vi "2. MotorTest.vi"(1 "Stop Button":bool, 8 "error in (no error)":errorcluster, 10 "Speed (PWM)":dbl(slide) scale=-100.0..100.0) -> (0 "error out":errorcluster, 2 "MotorEncoder (deg)":dbl)   [LabVIEW 2019, in "SJCube_KNRm.lvlib"]
uses:
  SJCube_KNRm.lvlib
panel:
  in  "Reset Counter":bool
  out "gearedMotorEncoder (deg)":dbl
  # "ATTENTION:\n\nDO THIS EXP. ONLY WHEN THE PENDULUM \nIS \"NOT\" INSTALLED"
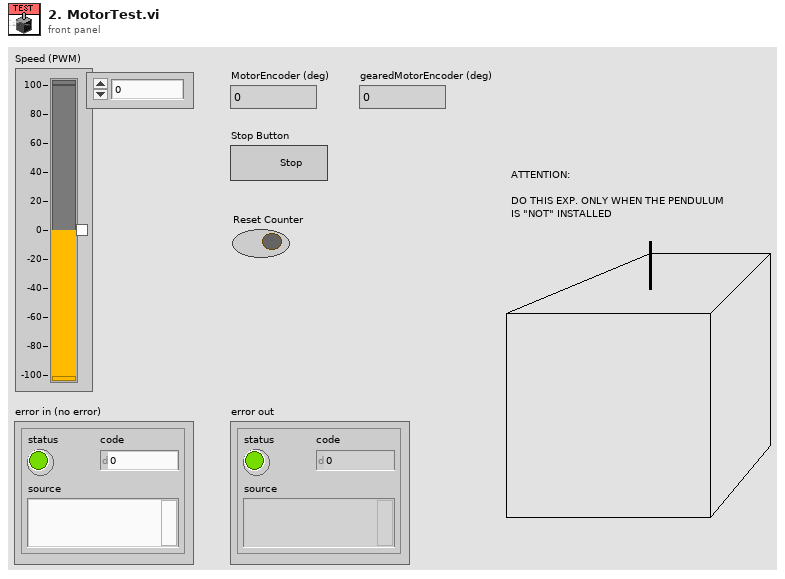
[diagram p1: front panel]
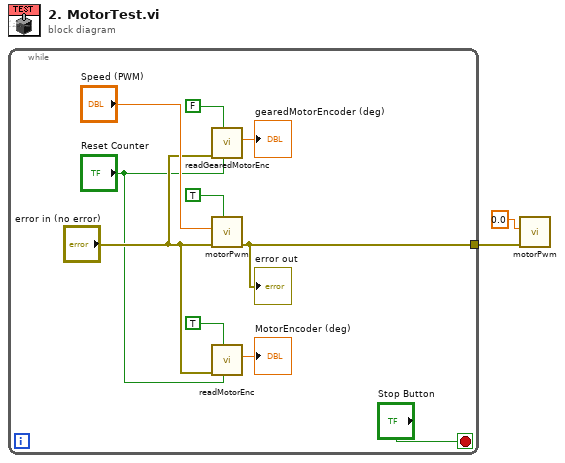
[diagram p0: block diagram]
diagram:
  n1 = while {
    tunnel: [w8] -> w2
    stop <- "Stop Button" stop-if-true
    n2 = call "readGearedMotorEnc.vi"("Reset Counter"="Reset Counter", "Reverse ENC?"=FALSE, "error in (no error)"="error in (no error)") -> ("gearedMotorEncoder (deg)"=→"gearedMotorEncoder (deg)":dbl)  [unwired: 7 in, 1 out]
    n3 = call "motorPwm.vi"("reverse?"=TRUE, "error in (no error)"="error in (no error)", "Speed (PWM)"="Speed (PWM)") -> ("error out"=w8:errorcluster)  [unwired: 8 in]
    "error out" <- w8
    n4 = call "readMotorEnc.vi"("Reset Counter"="Reset Counter", "Reverse ENC?"=TRUE, "error in (no error)"="error in (no error)") -> ("MotorEncoder (deg)"=→"MotorEncoder (deg)":dbl)  [unwired: 7 in, 1 out]
  }
  n5 = call "motorPwm.vi"("error in (no error)"=w2, "Speed (PWM)"=0.0) -> ()  [unwired: 9 in, 1 out]
